vi "File_Modified_Since_Check.vi"(1 "Pathname":path, 2 "Just Modified?":bool) -> (0 "Modified?":bool)   [LabVIEW 2010]
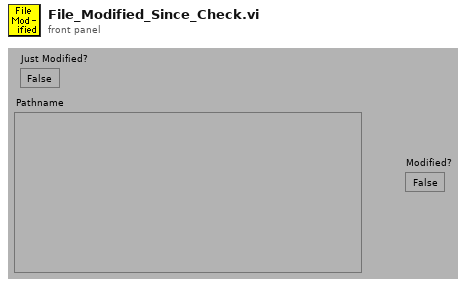
[diagram p1: front panel]
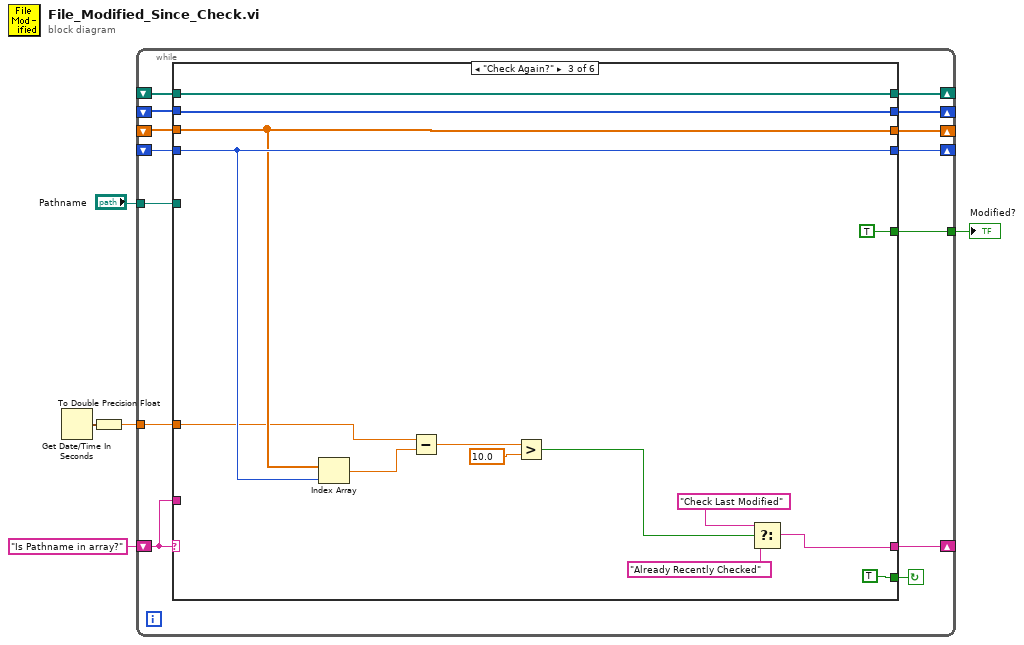
[diagram p0: block diagram]
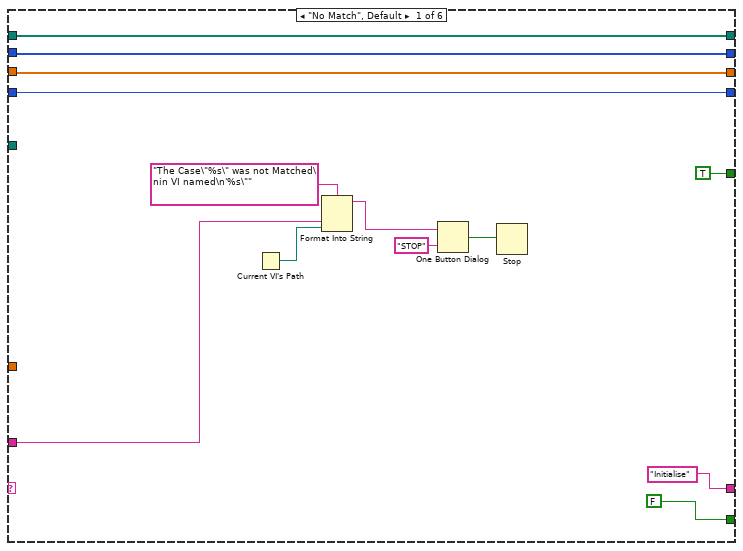
[diagram p2: hidden frame]
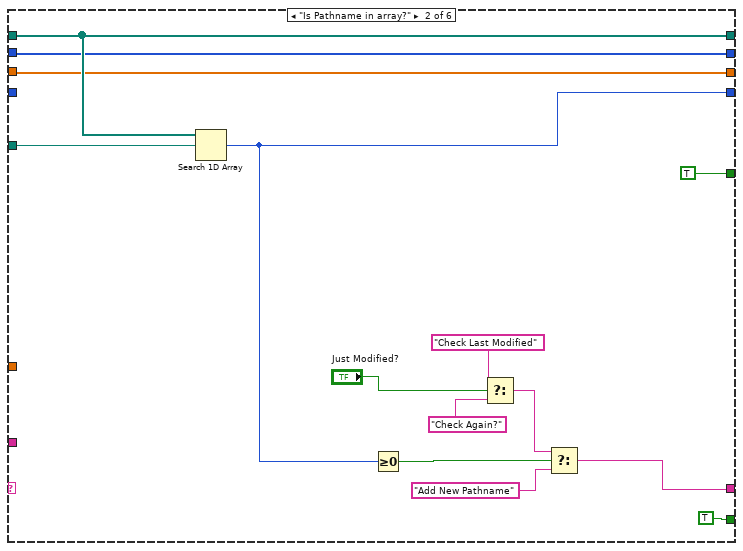
[diagram p3: hidden frame]
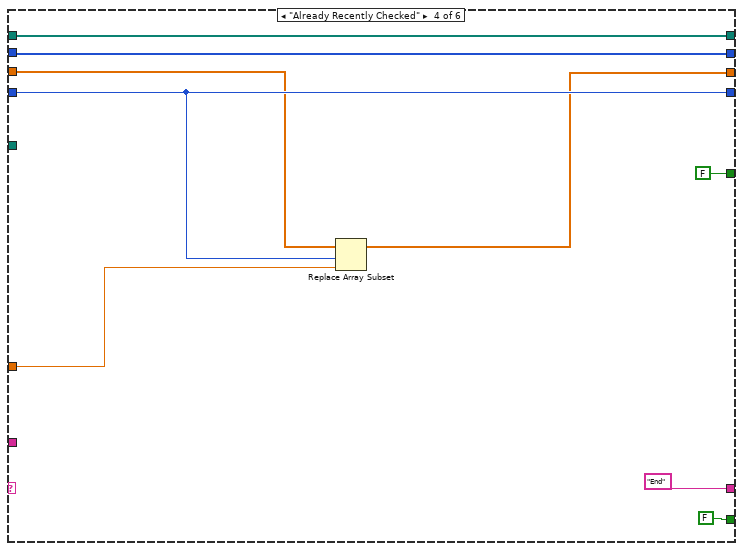
[diagram p4: hidden frame]
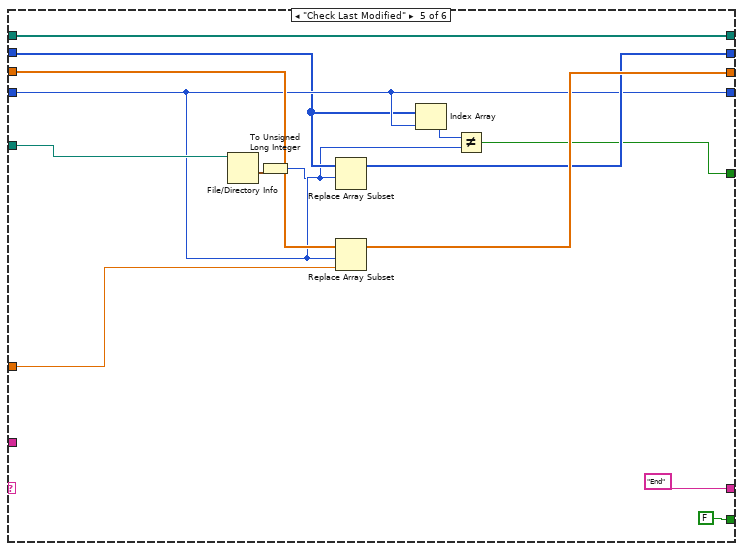
[diagram p5: hidden frame]
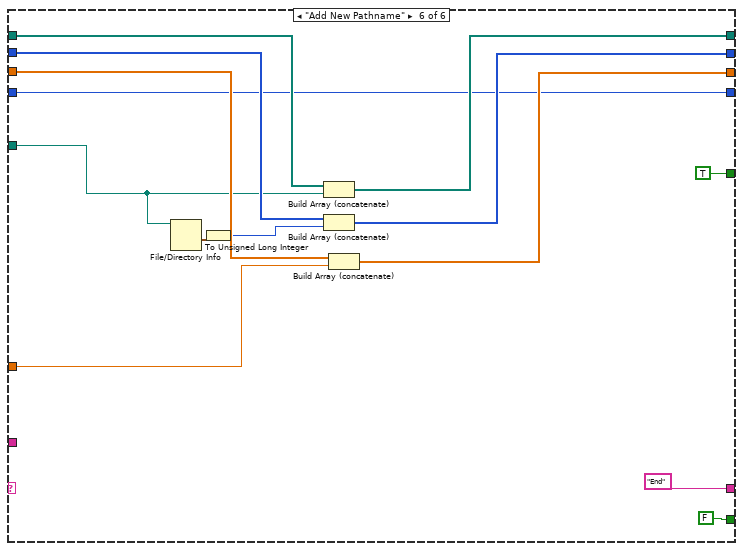
[diagram p6: hidden frame]
diagram:
  n1 = Get Date/Time In Seconds() -> (seconds since 1Jan1904=w1:timestamp)
  n2 = To Double Precision Float(number=w1) -> (double precision float=w4:dbl)
  n3 = while {
    tunnel: [w6] -> w3
    shift-left: _ -> [w10]
    shift-right: [w9] -> _
    tunnel: w4 -> [w11]
    tunnel: "Pathname" -> [w15]
    shift-left: _ -> [w13]
    shift-right: [w7] -> _
    shift-left: _ -> [w14]
    shift-right: [w8] -> _
    shift-left: _ -> [w16]
    shift-right: [w12] -> _
    shift-left: "Is Pathname in array?" ("f") -> [w17]
    shift-right: [w18] -> _
    stop <- w19 continue-if-true
    n4 = case shown="\"Check Again?\"" w17 {
      tunnel: [FALSE TRUE TRUE FALSE FALSE FALSE] -> w19
      tunnel: ["Initialise" w39 w49 "End" "End" "End"] -> w18
      tunnel: w17 -> [w27 _ _ _ _ _]
      tunnel: w16 -> [w24 w44 w59 w67 w81 w95]
      tunnel: w15 -> [_ w45 _ _ w77 w88]
      tunnel: w14 -> [w23 w43 w58 w66 w74 w94]
      tunnel: w13 -> [w22 w42 w55 w63 w79 w93]
      tunnel: [w24 w44 w59 w67 w81 w92] -> w12
      tunnel: w11 -> [_ _ w53 w64 w80 w89]
      tunnel: w10 -> [w21 _ w56 w65 w75 w86]
      tunnel: [w21 w41 w56 w65 w75 w86] -> w9
      tunnel: [w23 w43 w58 w66 w76 w91] -> w8
      tunnel: [w22 w42 w55 w62 w78 w90] -> w7
      tunnel: [TRUE TRUE TRUE FALSE w71 TRUE] -> w6
      frame "No Match", Default {
        n5 = Current VI's Path() -> (path=w26:path)
        n6 = Format Into String(format string="The Case\"%s\" was not Matched\nin VI named\n'%s\"" ("Format String"), w27, w26) -> (resulting string=w30:string)  [unwired: 2 in, 1 out]
        n7 = One Button Dialog(message=w30, button name ("OK")="STOP") -> (true=w28:bool)
        n8 = Stop(stop? (T)=w28) -> ()
      }
      frame "Is Pathname in array?" {
        n9 = Search 1D Array(1D array=w44, element=w45) -> (index of element=w41:i32)  [unwired: 1 out]
        n10 = Greater Or Equal To 0?(x=w41) -> (x >= 0?=w40:bool)
        n11 = Select(t="Check Last Modified", s="Just Modified?", f="Check Again?") -> (s? t:f=w33:string)
        n12 = Select(t=w33, s=w40, f="Add New Pathname") -> (s? t:f=w39:string)
      }
      frame "Check Again?" {
        n13 = Index Array(array=w55, index=w56) -> (element=w54:dbl)
        n14 = Subtract(x=w53, y=w54) -> (x-y=w52:dbl)
        n15 = Greater?(x=w52, y=10.0) -> (0:w48:bool)
        n16 = Select(t="Check Last Modified", s=w48, f="Already Recently Checked") -> (s? t:f=w49:string)
      }
      frame "Already Recently Checked" {
        n17 = Replace Array Subset(array=w63, new element=w64, index=w65) -> (w62:dbl[])
      }
      frame "Check Last Modified" {
        n18 = File/Directory Info(path=w77) -> (last mod=w70:timestamp)  [unwired: 1 in, 6 out]
        n19 = To Unsigned Long Integer(number=w70) -> (unsigned 32bit integer=w72:u32)
        n20 = Replace Array Subset(array=w74, new element=w72, index=w75) -> (w76:u32[])
        n21 = Replace Array Subset(array=w79, new element=w80, index=w75) -> (w78:dbl[])
        n22 = Index Array(array=w74, index=w75) -> (element=w73:u32)
        n23 = Not Equal?(x=w73, y=w72) -> (x != y?=w71:bool)
      }
      frame "Add New Pathname" {
        n24 = File/Directory Info(path=w88) -> (last mod=w84:timestamp)  [unwired: 1 in, 6 out]
        n25 = To Unsigned Long Integer(number=w84) -> (unsigned 32bit integer=w87:u32)
        n26 = Build Array (concatenate)(w95, w88) -> (w92:path[])
        n27 = Build Array (concatenate)(w94, w87) -> (w91:u32[])
        n28 = Build Array (concatenate)(w93, w89) -> (w90:dbl[])
      }
    }
  }
  "Modified?" <- w3
